vi "HEWH Standard Valve States.vi"(8 "Error In":errorcluster, 10 "Pressurize Tank?":bool, 11 "Valve Bank Setting":T3) -> (0 "Error Out":errorcluster, 1 "Drain/Purge Valve":T2="OFF", 2 "Outlet Valve":T1="OFF", 3 "Input Valve":T1="ON")   [LabVIEW 2016]
uses:
  Type Definitions/HEWH Valve Bank Positions.ctl
  Type Definitions/HEWH Normally Closed Valve Control.ctl
  Type Definitions/HEWH Normally Open Valve Control.ctl
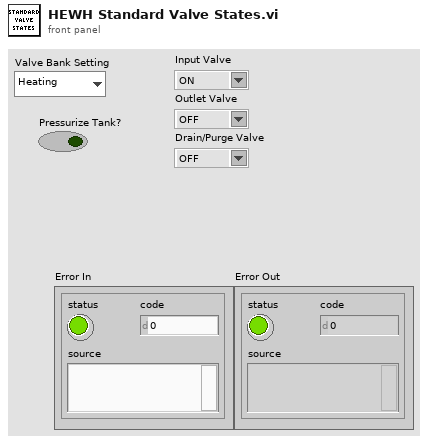
[diagram p1: front panel]
types:
  T1 = typedef "HEWH Normally Open Valve Control.ctl" = string
  T2 = typedef "HEWH Normally Closed Valve Control.ctl" = string
  T3 = typedef "HEWH Valve Bank Positions.ctl" = enum16{"Heating", "Purge", "Resting", "Draw"}
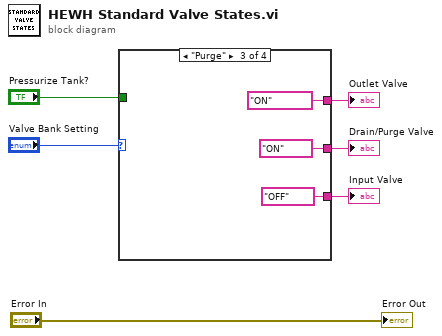
[diagram p0: block diagram]
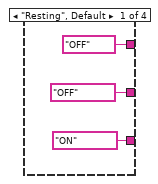
[diagram p2: hidden frame]
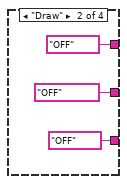
[diagram p3: hidden frame]
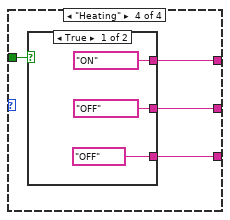
[diagram p4: hidden frame]
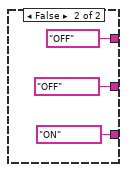
[diagram p5: hidden frame]
diagram:
  n1 = case shown="\"Purge\"" "Valve Bank Setting" {
    tunnel: "Pressurize Tank?" -> [_ _ _ w19]
    tunnel: [T2 "OFF" ("Drain/Purge Valve") T2 "OFF" ("Drain/Purge Valve") T2 "ON" ("Drain/Purge Valve") w18] -> w3
    tunnel: [T1 "OFF" ("Outlet Valve") T1 "OFF" ("Outlet Valve") T1 "ON" ("Outlet Valve") w17] -> w2
    tunnel: [T1 "ON" ("Input Valve") T1 "OFF" ("Input Valve") T1 "OFF" ("Input Valve") w16] -> w1
    frame "Resting", Default {
    }
    frame "Draw" {
    }
    frame "Purge" {
    }
    frame "Heating" {
      n2 = case shown="True" w19 {
        tunnel: [T2 "OFF" ("Drain/Purge Valve") T2 "OFF" ("Drain/Purge Valve")] -> w18
        tunnel: [T1 "ON" ("Outlet Valve") T1 "OFF" ("Outlet Valve")] -> w17
        tunnel: [T1 "OFF" ("Input Valve") T1 "ON" ("Input Valve")] -> w16
        frame True {
        }
        frame False {
        }
      }
    }
  }
  "Outlet Valve" <- w2
  "Input Valve" <- w1
  "Drain/Purge Valve" <- w3
  "Error Out" <- "Error In"
